vi "Power Qualtiy - 7.vi"() -> ()   [LabVIEW 2015]
uses:
  <vilib>/addons/Electrical Power/Basic/Measurement/RMS (N Channels).vi
  <vilib>/addons/Electrical Power/Basic/Measurement/Power (1 Channel).vi
  <vilib>/addons/Electrical Power/Basic/NI_EP_Basic.lvlib
panel:
  in  "stop":bool
  out "Power Factor":dbl[](array[numeric])
  out "IHD 7":dbl
  out "IHD 5":dbl
  out "IHD 3":dbl
  out "IHD 1":dbl
  out "Voltage Waveform":dynamicdata(graph)
  out "Current Waveform":dynamicdata(graph)
  out "Current":dbl(knob) scale=0.0..10.0
  out "Voltage":dbl(knob) scale=0.0..250.0
  out "THD":dbl
  out "Current Harmonics":dynamicdata(graph)
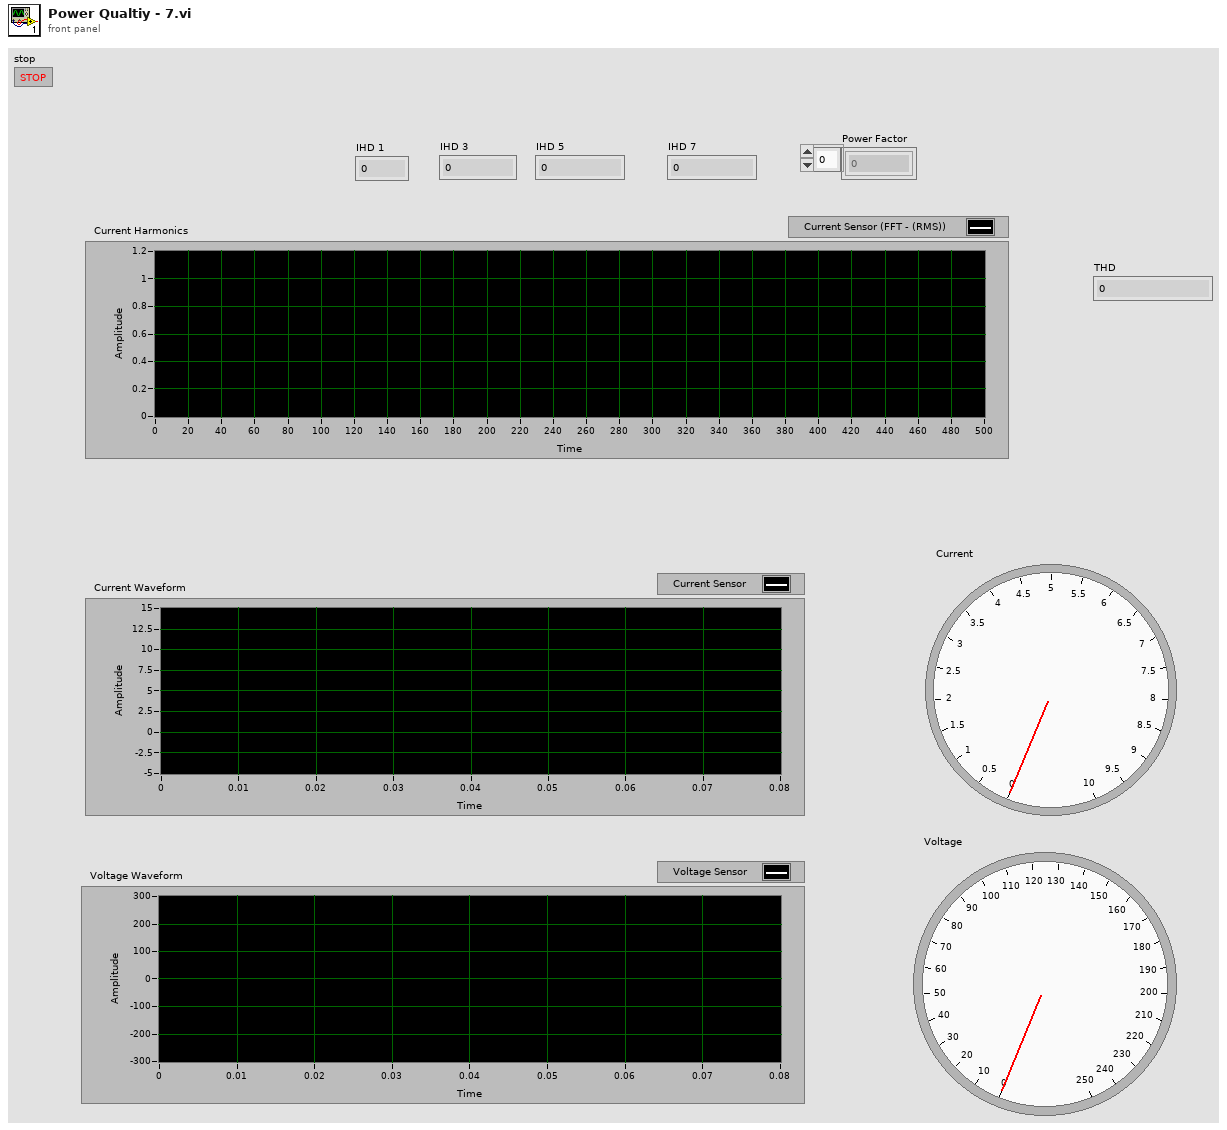
[diagram p1: front panel]
types:
  T1 = typedef "NI_EP_Basic.lvlib/basic_Power Value.ctl" = cluster{"active power [W]":dbl, "apparent power [VA]":dbl, "reactive power [VAR]":dbl, "power factor":dbl}
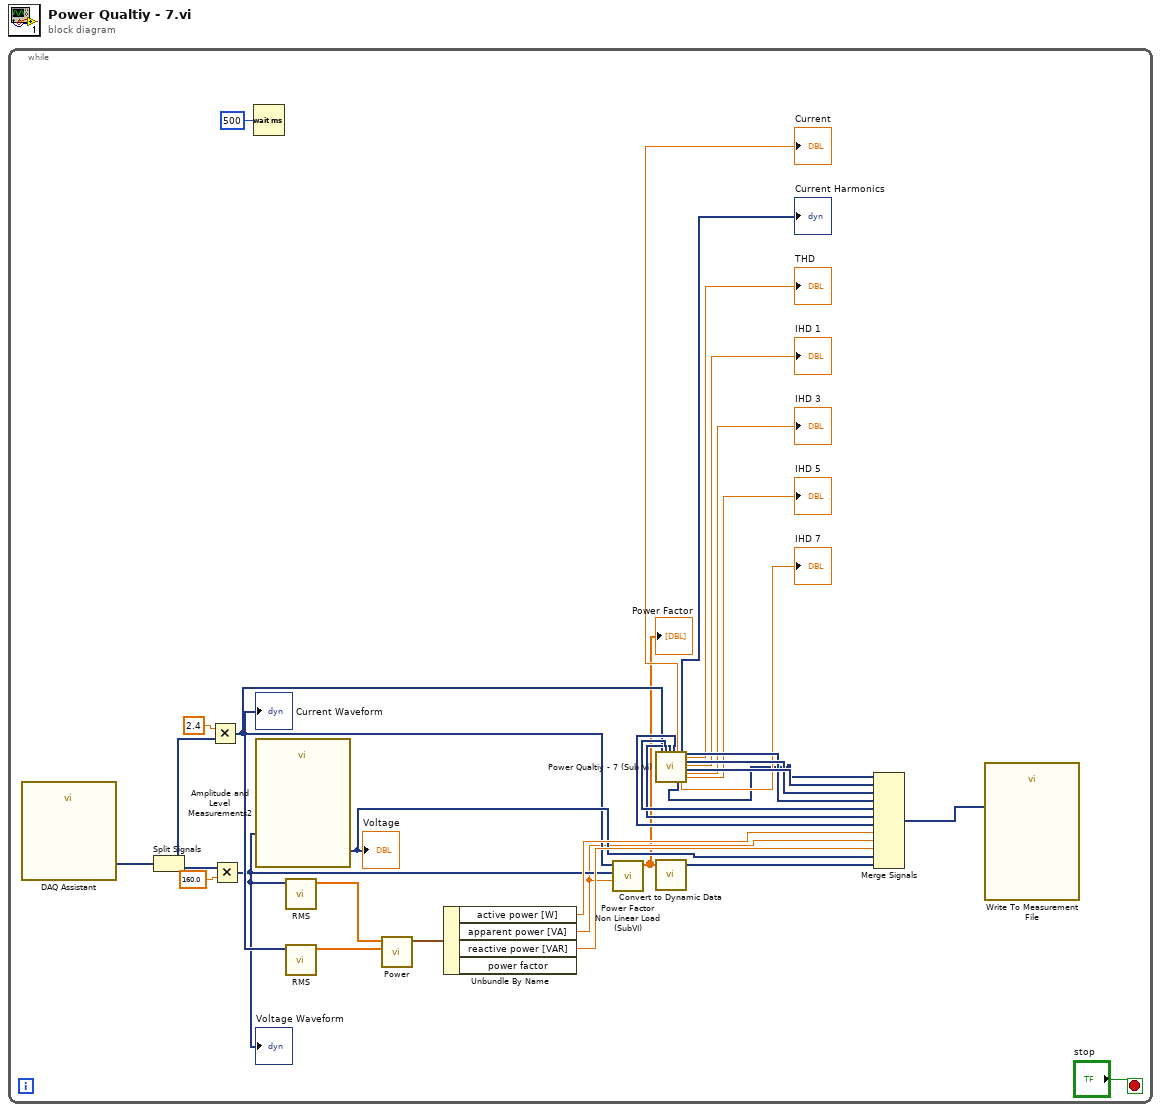
[diagram p0: block diagram]
diagram:
  n1 = while {
    stop <- "stop" stop-if-true
    n2 = call "DAQ Assistant"() -> ("data"=w33:dynamicdata)  [unwired: 17 in, 2 out]
    n3 = Split Signals(w33) -> (w32:dynamicdata, w31:dynamicdata)  [unwired: 2 in]
    n4 = Multiply(x=2.4, y=w32) -> (x*y=w9:dynamicdata)
    "Current Waveform" <- w9
    n5 = Multiply(x=w31, y=160.0) -> (x*y=w8:dynamicdata)
    "Voltage Waveform" <- w8
    n6 = Wait (ms)(milliseconds to wait=u32 500) -> ()  [unwired: 1 out]
    n7 = call "Amplitude and Level Measurements2"("Signals"=w8) -> ("RMS"=w10:dynamicdata)  [unwired: 13 in, 1 out]
    "Voltage" <- w10
    n8 = call-poly <vilib>:"RMS.vi"("waveforms"=w8) -> ("RMS values"=w28:dbl[])  [unwired: 9 in, 1 out]
    n9 = call-poly <vilib>:"RMS.vi"("waveforms"=w9) -> ("RMS values"=w27:dbl[])  [unwired: 9 in, 1 out]
    n10 = call-poly <vilib>:"Power.vi"("current waveform"=w27, "voltage waveform"=w28) -> ("power value"=w26:T1)  [unwired: 8 in, 1 out]
    n11 = Unbundle By Name(w26) -> ("active power [W]"=w19:dbl, "apparent power [VA]"=w7:dbl, "reactive power [VAR]"=w18:dbl)  [unwired: 1 out]
    n12 = call "Power Factor Non Linear Load (SubVI).vi"("apparent power [VA]"=w7, "Dynamic Data"=w8, "Dynamic Data 2"=w9) -> ("Power Factor"=w6:dbl[])  [unwired: 8 in]
    "Power Factor" <- w6
    n13 = call "Power Qualtiy - 7 (Sub Vi).vi"("Dynamic Data 6"=w9) -> ("Dynamic Data 2"=w21:dynamicdata, "Dynamic Data"=w20:dynamicdata, "Dynamic Data 4"=w23:dynamicdata, "Current"=→"Current":dbl, "RMS"=w3:dynamicdata, "Current Harmonics"=→"Current Harmonics":dynamicdata, "IHD 7"=→"IHD 7":dbl, "Dynamic Data 3"=w22:dynamicdata, "THD"=→"THD":dbl, "Dynamic Data 5"=w24:dynamicdata, "IHD 1"=→"IHD 1":dbl, "THD 2"=w25:dynamicdata, "IHD 3"=→"IHD 3":dbl, "IHD 5"=→"IHD 5":dbl)  [unwired: 12 in, 1 out]
    n14 = call "Convert to Dynamic Data"("Array"=w6) -> ("Dynamic Data Type"=w5:dynamicdata)  [unwired: 3 in]
    n15 = Merge Signals(w3, w25, w24, w22, w21, w20, w23, w19, w7, w18, w10, w5) -> (w4:dynamicdata)
    n16 = call "Write To Measurement File"("Signals"=w4) -> ()  [unwired: 16 in, 3 out]
  }
